vi "FRCts20_Backend_Competition_GET_return.vi"(7 "Competition":T1, 8 "error in (no error)":errorcluster, 11 "recordset data":variant[][](array[variant])) -> (0 "error out":errorcluster, 3 "data string":string)   [LabVIEW 2014]
uses:
  FRCts20_Backend_DBCluster_Competition_GET.ctl
  FRCts20_Backend_Engine.lvlib
  <vilib>/addons/database/_DB Variant To Data/Database Variant To Data.xnode
  FRCts20_Backend_API/FRCts20_Backend_API_Competition.ctl
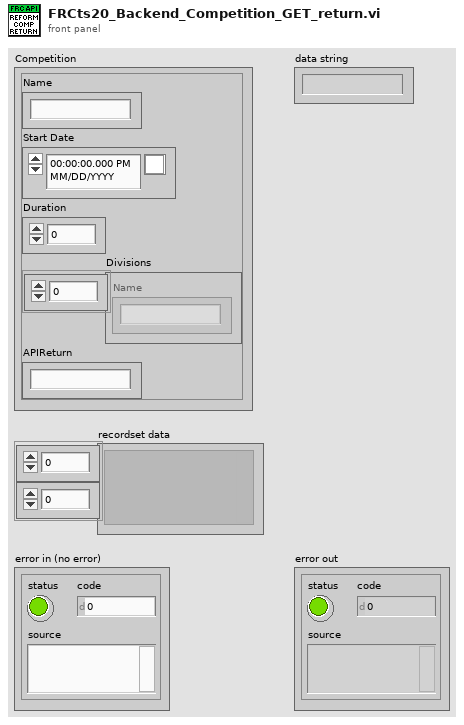
[diagram p1: front panel]
types:
  T1 = typedef "FRCts20_Backend_API.lvlib/FRCts20_Backend_API_Competition.ctl" = cluster{"Name":string, "Start Date":timestamp, "Duration":u8, "Divisions":string[], "APIReturn":string}
  T2 = typedef "FRCts20_Backend_Engine.lvlib/FRCts20_Backend_DBCluster_Competition_GET.ctl" = cluster{"StartTime":timestamp, "Duration":u8, "DivName":string}
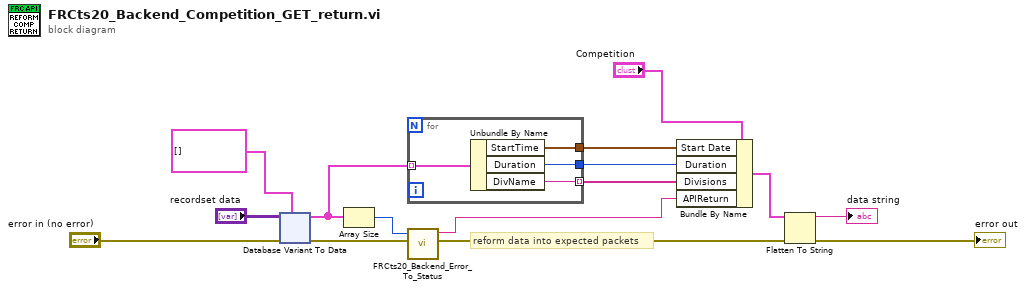
[diagram p0: block diagram]
diagram:
  # "reform data into expected packets"
  n1 = xnode "Database Variant To Data"("database variant"="recordset data", "error in"="error in (no error)", "type"=T2[] []) -> ("data"=w11:T2[], "error out"=w13:errorcluster)
  n2 = Array Size(array=w11) -> (size(s)=w5:i32)
  n3 = for {
    tunnel: [w19] -> w10
    tunnel: [w18] -> w9
    tunnel: [w17] -> w8 mode=indexing
    tunnel: w11 -> [w16] mode=indexing
    n4 = Unbundle By Name(w16) -> ("StartTime"=w19:timestamp, "Duration"=w18:u8, "DivName"=w17:string)
  }
  n5 = call "FRCts20_Backend_Error_To_Status.vi"("error in (no error)"=w13, "rows affected"=w5) -> ("error out"=w6:errorcluster, "String"=w7:string)  [unwired: 8 in]
  n6 = Bundle By Name(cluster="Competition", "Start Date"=w10, "Duration"=w9, "Divisions"=w8, "APIReturn"=w7) -> (w2:T1)
  n7 = Flatten To String(anything=w2, error in (no error)=w6) -> (data string=→"data string":string, error out=→"error out":errorcluster)  [unwired: 2 in, 1 out]
